vi "Periodic Timeout.vi"(6 "Now":u32, 9 "Period/Timeout":i32, 10 "Periodic Name":string, 11 "Module in":refnum<class "Module.lvclass">) -> (1 "Deadline":u32, 2 "Message":string, 3 "Module out":refnum<class "Module.lvclass">, 5 "Periodic":bool)   [LabVIEW 2023, in "Volatus.lvlib" / "Module.lvclass"]
uses:
  Module.lvclass
  Module.lvclass/Module.ctl
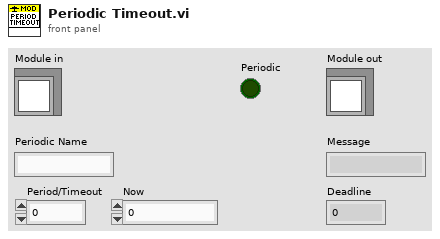
[diagram p1: front panel]
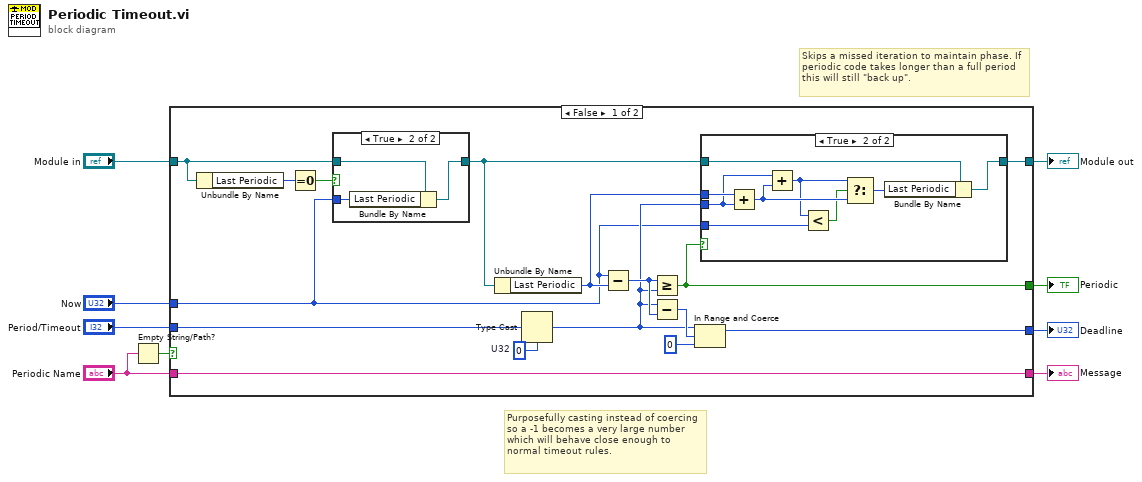
[diagram p0: block diagram]
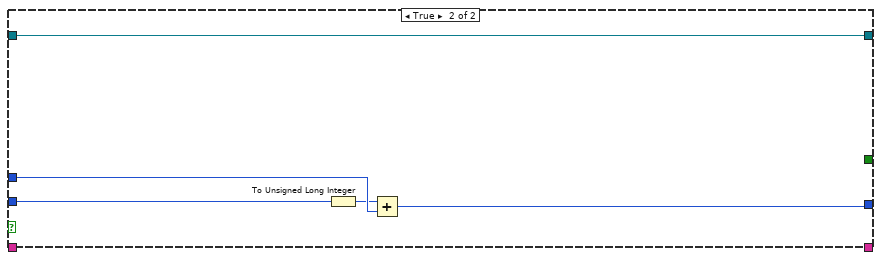
[diagram p4: hidden frame]
diagram:
  # "Skips a missed iteration to maintain phase. If periodic code takes longer than a full period this will still \"back up\"."
  # "Purposefully casting instead of coercing so a -1 becomes a very large number which will behave close enough to normal timeout rules."
  n1 = Empty String/Path?(string/path="Periodic Name") -> (empty?=w9:bool)
  n2 = case shown="False" w9 {
    tunnel: [w25 _] -> w8
    tunnel: "Periodic Name" -> [w25 _]
    tunnel: "Period/Timeout" -> [w24 w44]
    tunnel: [w20 w41] -> w5
    tunnel: "Now" -> [w14 w43]
    tunnel: "Module in" -> [w12 w40]
    tunnel: [w15 w40] -> w2
    tunnel: [w18 _] -> w1
    frame False {
      w23 = u32 0  # U32
      n3 = Unbundle By Name(w12) -> ("Last Periodic"=w11:u32)
      n4 = Equal To 0?(x=w11) -> (x = 0?=w10:bool)
      n5 = case shown="True" w10 {
        tunnel: w12 -> [w26 w29]
        tunnel: w14 -> [_ w28]
        tunnel: [w26 w27] -> w13
        frame False {
        }
        frame True {
          n6 = Bundle By Name(cluster=w29, "Last Periodic"=w28) -> (w27:refnum<class "Module.lvclass">)
        }
      }
      n7 = Unbundle By Name(w13) -> ("Last Periodic"=w17:u32)
      n8 = Type Cast(type=w23, x=w24) -> (*(type *) &x=w16:u32)
      n9 = Subtract(x=w14, y=w17) -> (x-y=w19:u32)
      n10 = Greater Or Equal?(x=w19, y=w16) -> (x >= y?=w18:bool)
      n11 = Subtract(x=w16, y=w19) -> (x-y=w22:u32)
      n12 = In Range and Coerce(upper limit=w16, x=w22, lower limit=u32 0) -> (coerced(x)=w20:u32)  [unwired: 1 out]
      n13 = case shown="True" w18 {
        tunnel: w13 -> [w30 w38]
        tunnel: w17 -> [_ w39]
        tunnel: w16 -> [_ w36]
        tunnel: [w30 w37] -> w15
        tunnel: w14 -> [_ w35]
        frame False {
        }
        frame True {
          n14 = Add(x=w39, y=w36) -> (x+y=w34:u32)
          n15 = Add(x=w36, y=w34) -> (x+y=w33:u32)
          n16 = Less?(x=w33, y=w35) -> (x < y?=w32:bool)
          n17 = Select(t=w33, s=w32, f=w34) -> (s? t:f=w31:u32)
          n18 = Bundle By Name(cluster=w38, "Last Periodic"=w31) -> (w37:refnum<class "Module.lvclass">)
        }
      }
    }
    frame True {
      n19 = To Unsigned Long Integer(number=w44) -> (unsigned 32bit integer=w42:u32)
      n20 = Add(x=w42, y=w43) -> (x+y=w41:u32)
    }
  }
  "Module out" <- w2
  "Deadline" <- w5
  "Message" <- w8
  "Periodic" <- w1
